vi "Stereo Vision - Corresponding Points Dialog.vi"(8 "error in (no error)":errorcluster, 10 "Right Image in":T1, 11 "Left Image in":T1) -> (0 "error out":errorcluster, 2 "Right Image out":T1, 3 "Left Image out":T1)   [LabVIEW 2014]
doc: "Lets the user specify corresponding points on the left and right images."
uses:
  <vilib>/vision/Image Controls.llb/IMAQ Image.ctl
  <vilib>/vision/NI_Vision_Development_Module.lvlib
panel:
  # "Overview: Set the calibration axis origin for both images as the top left point of the first left and right grids."
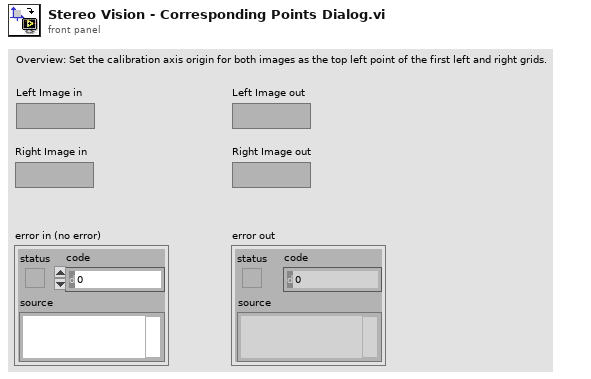
[diagram p1: front panel]
types:
  T1 = typedef "IMAQ Image.ctl" = refnum<image>
  T2 = cluster{"Origin Pixel":cluster{"X":sgl, "Y":sgl}, "Angle Relative to Horizontal (deg)":sgl, "Axis Reference":u32}
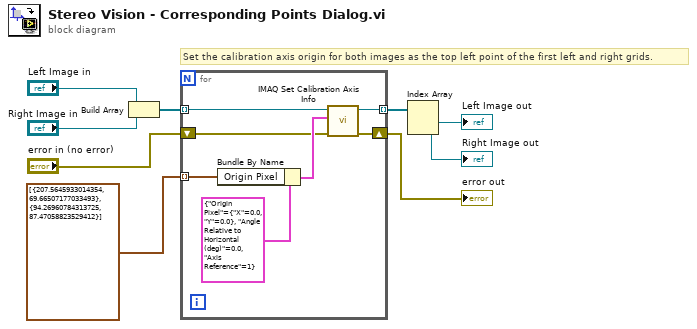
[diagram p0: block diagram]
diagram:
  # "Set the calibration axis origin for both images as the top left point of the first left and right grids."
  n1 = Build Array("Left Image in", "Right Image in") -> (w4:T1[])
  n2 = for {
    tunnel: w4 -> [w16] mode=indexing
    tunnel: cluster{"X":dbl, "Y":dbl}[] [{"X"=207.5645933014354, "Y"=69.66507177033493}, {"X"=94.26960784313725, "Y"=87.47058823529412}] ("appended array") -> [w14] mode=indexing
    tunnel: [w12] -> w5 mode=indexing
    shift-right: [w11] -> w7
    shift-left: "error in (no error)" -> [w10]
    n3 = Bundle By Name(cluster=T2 {"Origin Pixel"={"X"=0.0, "Y"=0.0}, "Angle Relative to Horizontal (deg)"=0.0, "Axis Reference"=1} ("Calibration Axis Info"), "Origin Pixel"=w14) -> (w13:T2)
    n4 = call "IMAQ Set Calibration Axis Info"("error in (no error)"=w10, "Calibration Axis Info"=w13, "Calibration Template Image In"=w16) -> ("error out"=w11:errorcluster, "Calibration Template Image Out"=w12:T1)  [unwired: 7 out]
  }
  "error out" <- w7
  n5 = Index Array(array=w5) -> (element #1=→"Left Image out":T1, element #2=→"Right Image out":T1)  [unwired: 2 in]
